vi "mod_Locate burst.vi"(0 "input complex waveform":T1 {"Y" format="%.3f"; "dt" format="%^.2e"; "t0" format="%.4f"}, 5 "burst duration (s)":dbl=-1.0 format="%.2p", 7 "trigger level (V)":dbl=0.01 format="%.2p", 9 "hysteresis":dbl format="%.2p", 11 "error in (no error)":errorcluster, 12 "reset ? (T)":bool=TRUE) -> (4 "output complex waveform":T1 {"Y" format="%.3f"; "dt" format="%^.2e"; "t0" format="%.4f"}, 6 "trigger detected?":bool, 8 "trigger location":i32, 15 "error out":errorcluster)   [LabVIEW 2020, in "niDMT.lvlib"]
uses:
  <vilib>/addons/Modulation/niDMT.lvlib
  <vilib>/addons/Modulation/Analog/controls/Complex Data Waveform.ctl
  <vilib>/measure/mamon.llb/Trigger Detection for 1 Channel (obs).vi
  <vilib>/addons/Modulation/niAMT.lvlib
  <vilib>/measure/NI_MAPro.lvlib
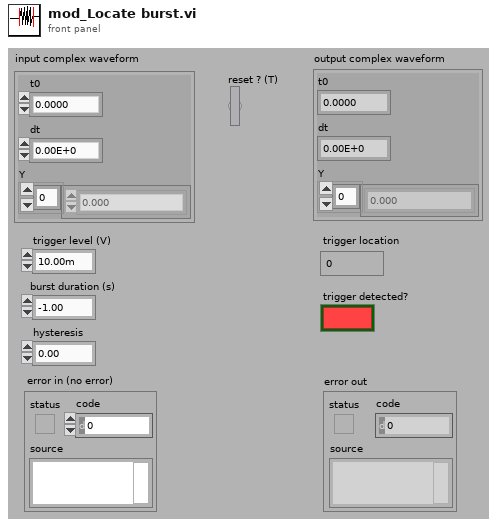
[diagram p1: front panel]
types:
  T1 = typedef "niAMT.lvlib/Complex Data Waveform.ctl" = cluster{"t0":dbl, "dt":dbl, "Y":cdb[]}
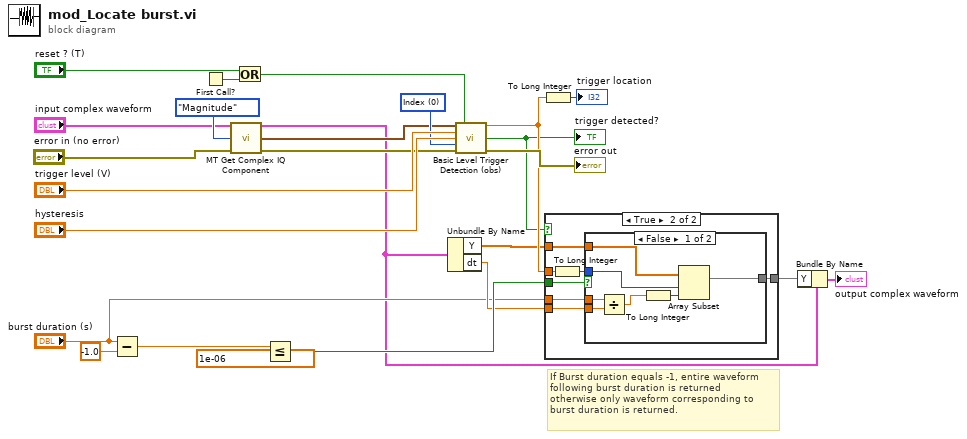
[diagram p0: block diagram]
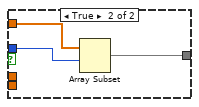
[diagram p3: hidden frame]
diagram:
  w23 = u16 0 items=["Index", "Time"] ("mode")
  # "If Burst duration equals -1, entire waveform\nfollowing burst duration is returned\notherwise only waveform corresponding to\nburst duration is returned."
  n1 = Subtract(x="burst duration (s)", y=-1.0) -> (x-y=w16:dbl)
  n2 = First Call?() -> (First Call?: T/F=w5:bool)
  n3 = call <vilib>:"MT Get Complex IQ Component.vi"("IQ data (complex) in"="input complex waveform", "component choice"=enum16{"I", "Q", "Magnitude", "Phase"}."Magnitude", "error in (no error)"="error in (no error)") -> ("IQ data (complex) out"=w1:cluster{"t0":dbl, "dt":dbl, "Y":cdb[]}, "CE component"=w20:waveform(dbl), "error out"=w3:errorcluster)  [unwired: 1 in, 9 out]
  n4 = Or(x="reset ? (T)", y=w5) -> (x .or. y?=w6:bool)
  n5 = Less Or Equal?(x=w16, y=1e-06) -> (x <= y?=w14:bool)
  n6 = Unbundle By Name(w1) -> ("Y"=w12:cdb[], "dt"=w10:dbl)
  n7 = call-poly <vilib>:"Basic Level Trigger Detection (obs).vi"("signal in"=w20, "reset"=w6, "level"="trigger level (V)", "hysteresis"="hysteresis", "location mode"=w23, "error in (no error)"=w3) -> ("trigger location"=w13:dbl, "trigger detected?"=w7:bool, "error out"=→"error out":errorcluster)  [unwired: 1 in, 6 out]
  "trigger detected?" <- w7
  n8 = To Long Integer(number=w13) -> (32bit integer=→"trigger location":i32)
  n9 = case shown="True" w7 {
    tunnel: w14 -> [_ w32]
    tunnel: w13 -> [_ w27]
    tunnel: w12 -> [_ w31]
    tunnel: [_ w30] -> w11
    tunnel: w10 -> [_ w29]
    tunnel: "burst duration (s)" -> [_ w28]
    frame False {
    }
    frame True {
      n10 = To Long Integer(number=w27) -> (32bit integer=w26:i32)
      n11 = case shown="False" w32 {
        tunnel: w26 -> [w33 w40]
        tunnel: w31 -> [w39 w42]
        tunnel: [w35 w41] -> w30
        tunnel: w29 -> [w38 _]
        tunnel: w28 -> [w37 _]
        frame False {
          n12 = Divide(x=w37, y=w38) -> (x/y=w36:dbl)
          n13 = To Long Integer(number=w36) -> (32bit integer=w34:i32)
          n14 = Array Subset(array=w39, index=w33, length=w34) -> (w35:cdb[])
        }
        frame True {
          n15 = Array Subset(array=w42, index=w40) -> (w41:cdb[])  [unwired: 1 in]
        }
      }
    }
  }
  n16 = Bundle By Name(cluster=w1, "Y"=w11) -> (→"output complex waveform":cluster{"t0":dbl, "dt":dbl, "Y":cdb[]})
